vi "RGB Color.vi"(8 "error in (no error)":errorcluster, 10 "Color":u32(colorbox), 11 "Color in":refnum<class "Color.lvclass">) -> (0 "error out":errorcluster, 3 "Color out":refnum<class "Color.lvclass">)   [LabVIEW 2014, in "Color.lvclass"]
doc: "Sets the color class according to a colorbox input, for determining the RGB color values of the class. Use Set Alpha property separately if you want transparency."
uses:
  Color.lvclass
  System.Drawing
  Color.lvclass/Color.ctl
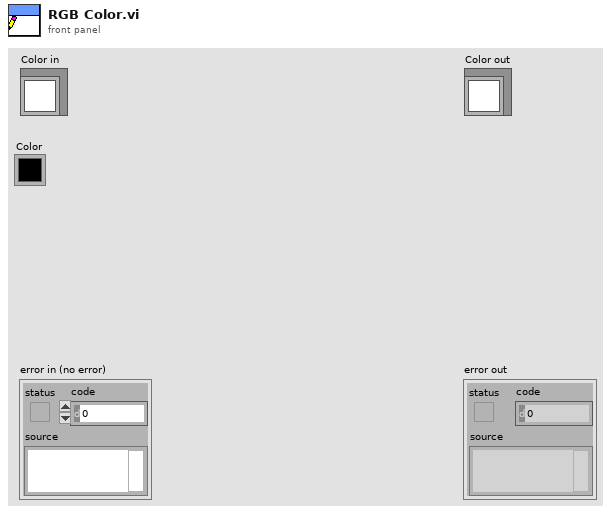
[diagram p1: front panel]
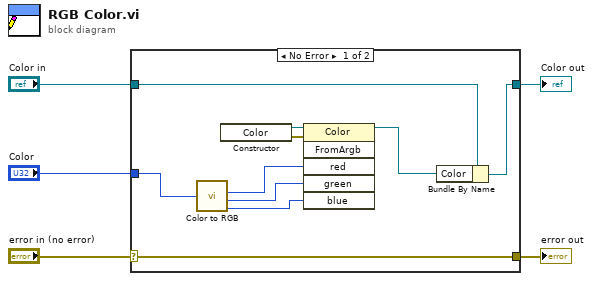
[diagram p0: block diagram]
diagram:
  n1 = case shown="No Error" "error in (no error)" {
    selector: "error in (no error)" -> [w15 w16]
    tunnel: [w15 w16] -> w4
    tunnel: [w13 w17] -> w2
    tunnel: "Color in" -> [w14 w17]
    tunnel: "Color" -> [w10 _]
    frame No Error {
      n2 = call <vilib>:"Color to RGB.vi"("Color"=w10) -> ("R"=w8:u8, "G"=w7:u8, "B"=w6:u8)  [unwired: 1 out]
      n3 = constructor class="Color"() -> (reference out=w12:refnum<k24>, error out=w11:errorcluster)  [unwired: 3 in, 1 out]
      n4 = invoke class="Color" method="FromArgb"(reference=w12, error in=w11, "red"=w8, "green"=w7, "blue"=w6) -> (reference out=w9:refnum<k24>)  [unwired: 1 in, 5 out]
      n5 = Bundle By Name(cluster=w14, "Color"=w9) -> (w13:refnum<class "Color.lvclass">)
    }
    frame Error {
    }
  }
  "error out" <- w4
  "Color out" <- w2
